vi "Load_And_Intitiate_Velocity.vi"(8 "Error In":errorcluster, 9 "Velocity":i16, 10 "Node":u8, 11 "Serial In":refnum<visa-resource-name>) -> (0 "Error Out":errorcluster, 3 "Serial Out":refnum<visa-resource-name>)   [LabVIEW 2019]
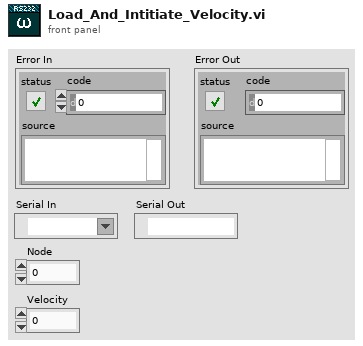
[diagram p1: front panel]
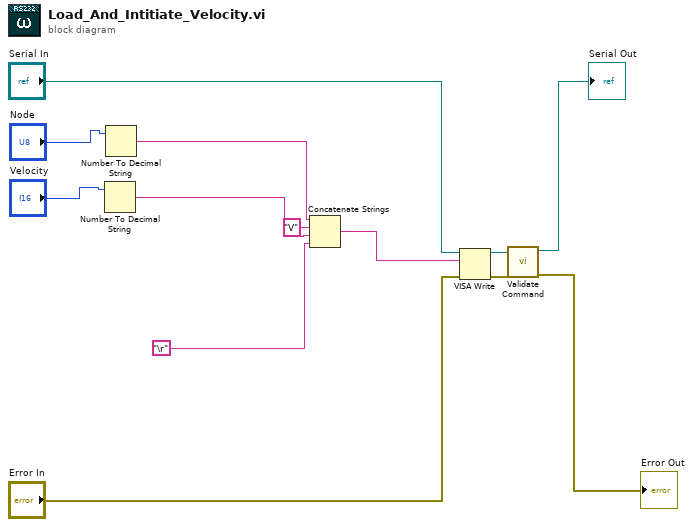
[diagram p0: block diagram]
diagram:
  n1 = Number To Decimal String(number="Velocity") -> (decimal integer string=w8:string)  [unwired: 1 in]
  n2 = Number To Decimal String(number="Node") -> (decimal integer string=w9:string)  [unwired: 1 in]
  n3 = Concatenate Strings(w9, "V" ("string"), w8, "\r") -> (w7:string)
  n4 = VISA Write(VISA resource name="Serial In", write buffer=w7, error in (no error)="Error In") -> (VISA resource name out=w4:refnum<visa-resource-name>, error out=w2:errorcluster)  [unwired: 1 out]
  n5 = call "Validate Command.vi"("error in (no error)"=w2, "Serial in"=w4) -> ("error out"=→"Error Out":errorcluster, "Serial Out"=→"Serial Out":refnum<visa-resource-name>)  [unwired: 3 in, 1 out]
